vi "FTW-CodeGen-Initialize.vi"(5 "XRef":refnum<vi>, 7 "Items":i32=3) -> (4 "State Out":T1)   [LabVIEW 2015, in "FTW-Dataflow-Synchronizer.xnode"]
uses:
  FTW-Dataflow-Synchronizer.xnode
  FTW-CodeGen-State.ctl
panel:
  # "Inputs"
  # "Outputs"
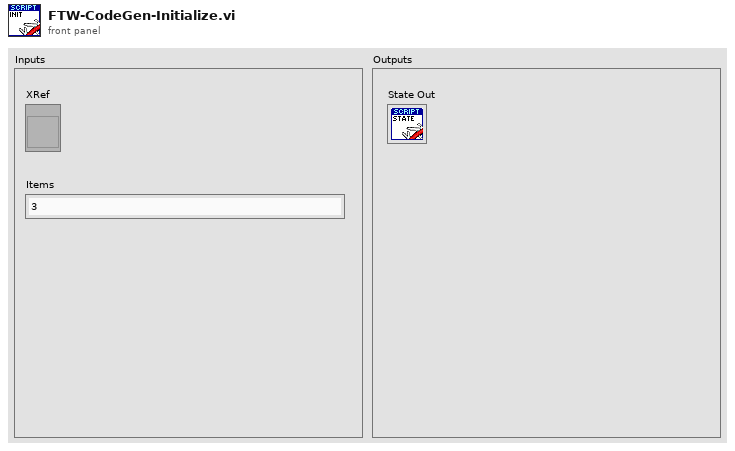
[diagram p1: front panel]
types:
  T1 = typedef "FTW-Dataflow-Synchronizer.xnode/FTW-CodeGen-State.ctl" = cluster{"InputTerminals":cluster{"Wired?":bool, "ID":string, "DataName":string, "DataColor":u32, "Type":variant}[], "EnableTiming?":bool}
  T2 = cluster{"Wired?":bool, "ID":string, "DataName":string, "DataColor":u32, "Type":variant}
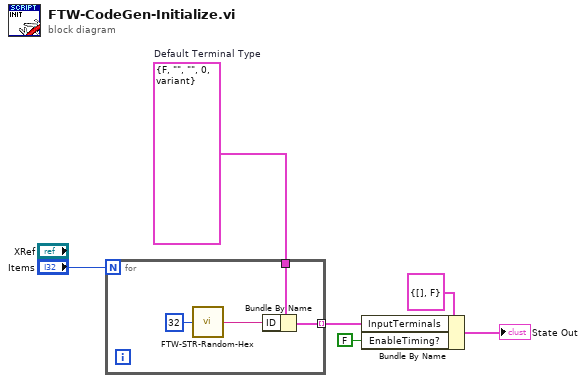
[diagram p0: block diagram]
diagram:
  w2 = T2 {"Wired?"=FALSE, "ID"="", "DataName"="", "DataColor"=0, "Type"=variant(variant variant)}  # Default Terminal Type
  n1 = for {
    N: "Items" -> [_]
    tunnel: [w9] -> w3 mode=indexing
    tunnel: w2 -> [w10]
    n2 = call "FTW-STR-Random-Hex.vi"("String Length"=32) -> ("Random Hex String"=w8:string)  [unwired: 3 in]
    n3 = Bundle By Name(cluster=w10, "ID"=w8) -> (w9:T2)
  }
  n4 = Bundle By Name(cluster=T1 {"InputTerminals"=[], "EnableTiming?"=FALSE} ("State Out"), "InputTerminals"=w3, "EnableTiming?"=FALSE) -> (→"State Out":T1)
